vi "CC Launch Quad Viewer.vi"(8 "error in (no error)":errorcluster, 11 "Files":path[](array[path])) -> (0 "error out":errorcluster, 3 "reference out":refnum<vi>)   [LabVIEW 2024]
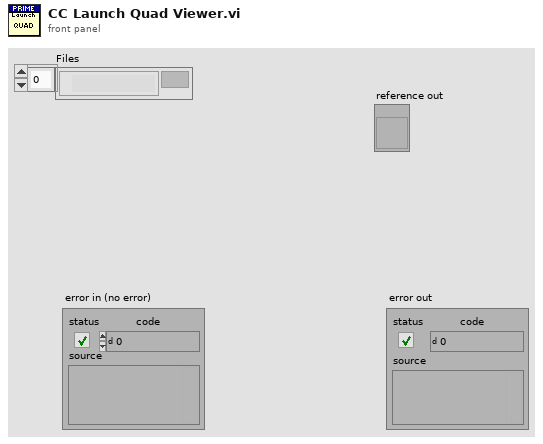
[diagram p1: front panel]
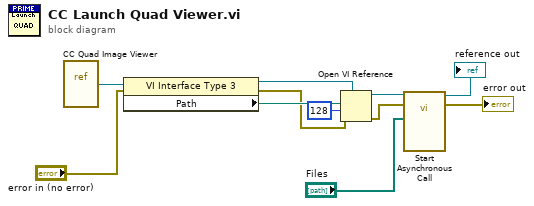
[diagram p0: block diagram]
diagram:
  n1 = vi-ref "CC Quad Image Viewer.vi"() -> (w11:refnum<vi>)
  n2 = property class="VI Interface Type 3"(reference=w11, error in="error in (no error)") -> (reference out=w9:refnum<vi>, error out=w4:errorcluster, "Path"=w10:path)
  n3 = Open VI Reference(type specifier VI Refnum (for type only)=w9, vi path=w10, options=128, error in (no error)=w4) -> (vi reference=w8:refnum<vi>, error out=w6:errorcluster)  [unwired: 2 in]
  n4 = call-by-ref "Start Asynchronous Call"(reference=w8, error in=w6, "Files"="Files") -> (reference out=→"reference out":refnum<vi>, error out=→"error out":errorcluster)  [unwired: 11 in]
